vi "dfd_SCL_ARMAOneMm_CU.vi"(8 "load":bool, 9 "global reset":bool, 11 "idx":u8) -> (3 "control signal":T1)   [LabVIEW 2017]
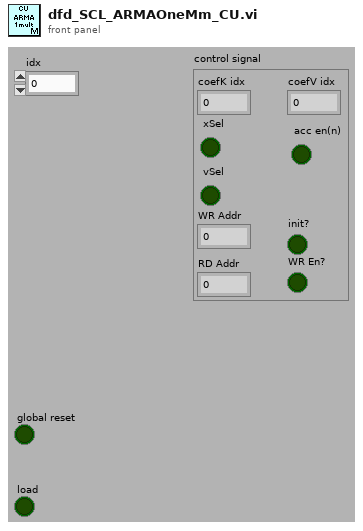
[diagram p1: front panel]
types:
  T1 = cluster{"coefK idx":u8, "coefV idx":u8, "xSel":bool, "vSel":bool, "acc en(n)":bool, "WR Addr":u16, "RD Addr":u16, "init?":bool, "WR En?":bool}
  T2 = cluster{"coefK idx":u8, "coefV idx":u8, "xSel ctrl(n)":bool, "xSel ctrl(n-1)":bool, "loop ctrl(n)":bool, "loop ctrl(n-1)":bool, "ySumSel ctrl(n)":bool, "ySumSel ctrl(n-1)":bool, "ySumSel ctrl(n-2)":bool, "ySumSel ctrl(n-3)":bool}
  T3 = cluster{"MEM RD Addr":u16, "MEM WR Addr":u16, "Ch cnt":u8, "first run?":bool}
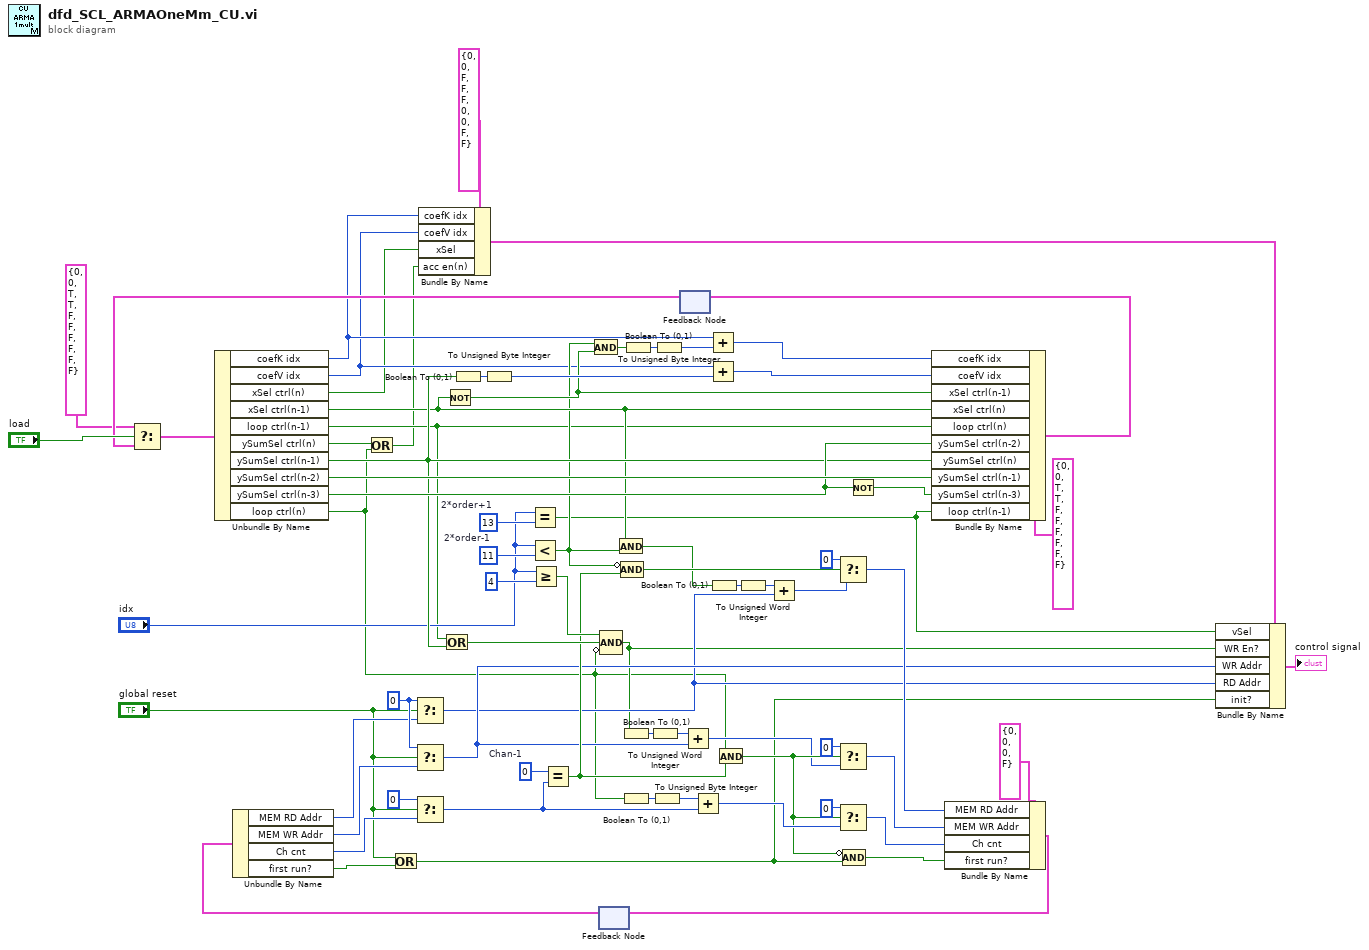
[diagram p0: block diagram]
diagram:
  w54 = u8 0  # Chan-1
  w62 = u16 0
  w67 = u8 11  # 2*order-1
  w70 = u8 13  # 2*order+1
  n1 = Equal?(x="idx", y=w70) -> (x = y?=w1:bool)
  n2 = Less?(x="idx", y=w67) -> (x < y?=w36:bool)
  n3 = Greater Or Equal?(x="idx", y=u8 4) -> (x >= y?=w41:bool)
  n4 = feedback #1() -> (w27:T3)  [unwired: 1 out]
  n5 = Unbundle By Name(w27) -> ("MEM RD Addr"=w60:u16, "MEM WR Addr"=w59:u16, "Ch cnt"=w58:u8, "first run?"=w56:bool)
  n6 = Or(x="global reset", y=w56) -> (x .or. y?=w14:bool)
  n7 = Select(t=w62, s="global reset", f=w60) -> (s? t:f=w15:u16)
  n8 = Select(t=w62, s="global reset", f=w59) -> (s? t:f=w16:u16)
  n9 = Select(t=u8 0, s="global reset", f=w58) -> (s? t:f=w51:u8)
  n10 = Equal?(x=w54, y=w51) -> (x = y?=w35:bool)
  n11 = Compound Arithmetic op=AND(invert w36, w35) -> (w34:bool)
  n12 = feedback #2() -> (w22:T2)  [unwired: 1 out]
  n13 = Select(t=T2 {"coefK idx"=0, "coefV idx"=0, "xSel ctrl(n)"=TRUE, "xSel ctrl(n-1)"=TRUE, "loop ctrl(n)"=FALSE, "loop ctrl(n-1)"=FALSE, "ySumSel ctrl(n)"=FALSE, "ySumSel ctrl(n-1)"=FALSE, "ySumSel ctrl(n-2)"=FALSE, "ySumSel ctrl(n-3)"=FALSE} ("control state out"), s="load", f=w22) -> (s? t:f=w21:T2)
  n14 = Unbundle By Name(w21) -> ("coefK idx"=w9:u8, "coefV idx"=w8:u8, "xSel ctrl(n)"=w7:bool, "xSel ctrl(n-1)"=w37:bool, "loop ctrl(n-1)"=w6:bool, "ySumSel ctrl(n)"=w5:bool, "ySumSel ctrl(n-1)"=w44:bool, "ySumSel ctrl(n-2)"=w72:bool, "ySumSel ctrl(n-3)"=w71:bool, "loop ctrl(n)"=w4:bool)
  n15 = Or(x=w5, y=w4) -> (x .or. y?=w3:bool)
  n16 = Bundle By Name(cluster=T1 {"coefK idx"=0, "coefV idx"=0, "xSel"=FALSE, "vSel"=FALSE, "acc en(n)"=FALSE, "WR Addr"=0, "RD Addr"=0, "init?"=FALSE, "WR En?"=FALSE} ("control signal"), "coefK idx"=w9, "coefV idx"=w8, "xSel"=w7, "acc en(n)"=w3) -> (w2:T1)
  n17 = Or(x=w6, y=w44) -> (x .or. y?=w42:bool)
  n18 = Not(x=w37) -> (.not. x?=w66:bool)
  n19 = Boolean To (0,1)(Boolean=w44) -> (0, 1=w69:i16)
  n20 = To Unsigned Byte Integer(number=w69) -> (unsigned 8bit integer=w68:u8)
  n21 = And(x=w36, y=w66) -> (x .and. y?=w64:bool)
  n22 = Compound Arithmetic op=AND(w41, w42, invert w4) -> (w13:bool)
  n23 = And(x=w37, y=w36) -> (x .and. y?=w28:bool)
  n24 = Boolean To (0,1)(Boolean=w13) -> (0, 1=w39:i16)
  n25 = Boolean To (0,1)(Boolean=w4) -> (0, 1=w53:i16)
  n26 = Boolean To (0,1)(Boolean=w64) -> (0, 1=w65:i16)
  n27 = To Unsigned Word Integer(number=w39) -> (unsigned 16bit integer=w40:u16)
  n28 = To Unsigned Byte Integer(number=w53) -> (unsigned 8bit integer=w52:u8)
  n29 = To Unsigned Byte Integer(number=w65) -> (unsigned 8bit integer=w63:u8)
  n30 = Add(x=w40, y=w16) -> (x+y=w38:u16)
  n31 = Add(x=w52, y=w51) -> (x+y=w49:u8)
  n32 = Add(x=w9, y=w63) -> (x+y=w12:u8)
  n33 = Add(x=w8, y=w68) -> (x+y=w11:u8)
  n34 = Boolean To (0,1)(Boolean=w28) -> (0, 1=w30:i16)
  n35 = And(x=w4, y=w35) -> (x .and. y?=w46:bool)
  n36 = To Unsigned Word Integer(number=w30) -> (unsigned 16bit integer=w29:u16)
  n37 = Add(x=w29, y=w15) -> (x+y=w32:u16)
  n38 = Select(t=u16 0, s=w34, f=w32) -> (s? t:f=w31:u16)
  n39 = Select(t=u16 0, s=w46, f=w38) -> (s? t:f=w45:u16)
  n40 = Select(t=u8 0, s=w46, f=w49) -> (s? t:f=w48:u8)
  n41 = Compound Arithmetic op=AND(invert w46, w14) -> (w55:bool)
  n42 = Not(x=w71) -> (.not. x?=w73:bool)
  n43 = Bundle By Name(cluster=T2 {"coefK idx"=0, "coefV idx"=0, "xSel ctrl(n)"=TRUE, "xSel ctrl(n-1)"=TRUE, "loop ctrl(n)"=FALSE, "loop ctrl(n-1)"=FALSE, "ySumSel ctrl(n)"=FALSE, "ySumSel ctrl(n-1)"=FALSE, "ySumSel ctrl(n-2)"=FALSE, "ySumSel ctrl(n-3)"=FALSE} ("control state out"), "coefK idx"=w12, "coefV idx"=w11, "xSel ctrl(n-1)"=w66, "xSel ctrl(n)"=w37, "loop ctrl(n)"=w6, "ySumSel ctrl(n-2)"=w71, "ySumSel ctrl(n)"=w44, "ySumSel ctrl(n-1)"=w72, "ySumSel ctrl(n-3)"=w73, "loop ctrl(n-1)"=w1) -> (w24:T2)
  n44 = feedback-in #2(w24) -> ()
  n45 = Bundle By Name(cluster=T3 {"MEM RD Addr"=0, "MEM WR Addr"=0, "Ch cnt"=0, "first run?"=FALSE} ("counter state in"), "MEM RD Addr"=w31, "MEM WR Addr"=w45, "Ch cnt"=w48, "first run?"=w55) -> (w25:T3)
  n46 = feedback-in #1(w25) -> ()
  n47 = Bundle By Name(cluster=w2, "vSel"=w1, "WR En?"=w13, "WR Addr"=w16, "RD Addr"=w15, "init?"=w14) -> (→"control signal":T1)
